vi "Undertake Command.vi"(0 "Operation":T1, 1 "Setpoint":dbl, 3 "Command Info In":T2, 4 "Description":string) -> (10 "Command Info Out":T2)   [LabVIEW 2023]
doc: "This template is useful for immediate subsystem actions that do not need deadband filtering\n\nBe sure to right-click and select New from Template and save with a new command name."
uses:
  <vilib>/Rock Robotics/WPI/Framework/Command Status Info.ctl
  <vilib>/Rock Robotics/WPI/Framework/Completion Status.ctl
  <vilib>/Rock Robotics/WPI/Framework/Completion Notifier.ctl
  Implementation/Undertake Operations.ctl
  Implementation/Undertake Setpoints.ctl
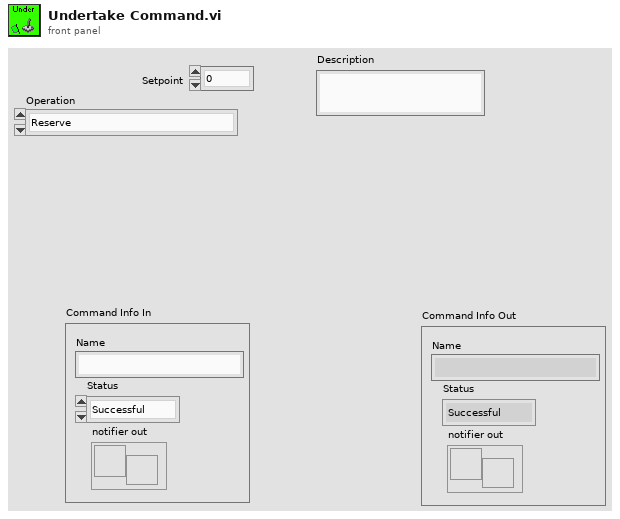
[diagram p1: front panel]
types:
  T1 = typedef "Undertake Operations.ctl" = enum16{"Reserve", "Read Current", "Immediate", "Onn", "Offf", "Reject"}
  T2 = typedef "Command Status Info.ctl" = cluster{"Name":string, "Status":T3, "notifier out":T4}
  T3 = typedef "Completion Status.ctl" = enum16{"Successful", "Aborted", "Incomplete"}
  T4 = typedef "Completion Notifier.ctl" = refnum<notifier>
  T5 = typedef "Undertake Setpoints.ctl" = cluster{"Operation":T1, "Speed":dbl}
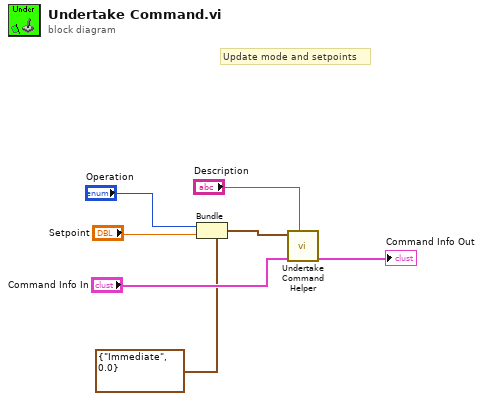
[diagram p0: block diagram]
diagram:
  # "Update mode and setpoints"
  n1 = Bundle(cluster=T5 {"Operation"=enum."Immediate", "Speed"=0.0} ("SubSystem Data"), "Operation"="Operation", "Speed"="Setpoint") -> (w2:T5)
  n2 = call "Undertake Command Helper.vi"("Description"="Description", "Command Info In"="Command Info In", "SubSystem Data"=w2) -> ("Command Info Out"=→"Command Info Out":T2)  [unwired: 6 in, 2 out]
